vi "addDataI64.vi"(8 "error in (no error)":errorcluster, 10 "Data":i64, 11 "FrameBuilder in":refnum<class "FrameBuilder.lvclass">) -> (0 "error out":errorcluster, 3 "FrameBuilder out":refnum<class "FrameBuilder.lvclass">)   [LabVIEW 2015, in "FrameBuilder.lvclass"]
uses:
  FrameBuilder.lvclass
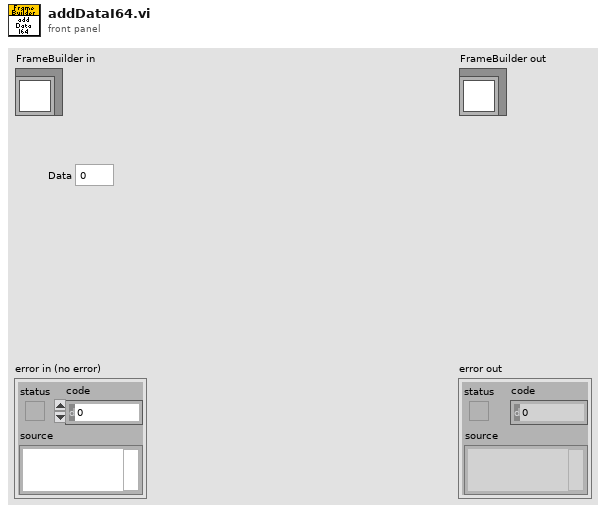
[diagram p1: front panel]
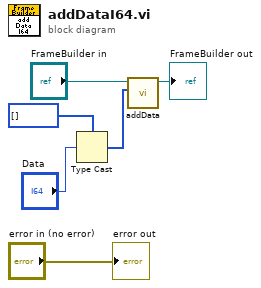
[diagram p0: block diagram]
diagram:
  n1 = Type Cast(type=u8[] [], x="Data") -> (*(type *) &x=w2:u8[])
  n2 = call "addData.vi"("Data"=w2, "FrameBuilder in"="FrameBuilder in") -> ("FrameBuilder out"=→"FrameBuilder out":refnum<class "FrameBuilder.lvclass">)  [unwired: 8 in, 1 out]
  "error out" <- "error in (no error)"
